vi "PlugIn Encoder.vi"(6 "String Value":string, 10 "Channel":T2, 11 "Menu":T1=enum."set reset") -> ()   [LabVIEW 2019]
uses:
  <vilib>/Rock Robotics/SystemInterfaces/Encoder/FPGA_EncoderIdx.ctl
  Encoder Update Ops.ctl
panel:
  # "Don't place this VI anywhere\nin your API code. It needs to\nbe a dynamically loaded\nwrapper of the main global"
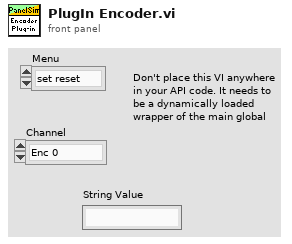
[diagram p1: front panel]
types:
  T1 = typedef "Encoder Update Ops.ctl" = enum16{"set init", "set count", "set period", "set reset", "set samples_to_avg", "get", "delete", "JSON update", "set name", "transmit initial", "reset", "set channel_a", "set channel_b"}
  T2 = typedef "FPGA_EncoderIdx.ctl" = enum8{"Enc 0", "Enc 1", "Enc 2", "Enc 3", "Enc 4", "Enc 5", "Enc 6", "Enc 7", "Invalid"}
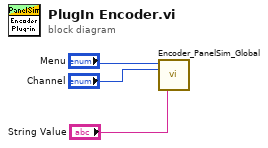
[diagram p0: block diagram]
diagram:
  n1 = call "Encoder_PanelSim_Global.vi"("menu"="Menu", "EncoderIndex"="Channel", "String Value"="String Value") -> ()  [unwired: 11 in, 2 out]
